vi "prima_apl_v0.vi"() -> ()   [LabVIEW 2009]
panel:
  out "Array":bool[](array[boolean])
  out "Numeric 8":dbl
  out "Numeric 7":dbl
  out "Numeric 6":dbl
  out "Numeric 5":dbl
  out "Numeric 4":dbl
  out "Numeric 3":dbl
  out "Numeric 2":dbl
  out "Numeric1":dbl
  out "Boolean 8":bool
  out "Boolean 7":bool
  out "Boolean 6":bool
  out "Boolean 5":bool
  out "Boolean 4":bool
  out "Boolean 3":bool
  out "Boolean 2":bool
  out "Boolean1":bool
  in  "Numeric 9":u8
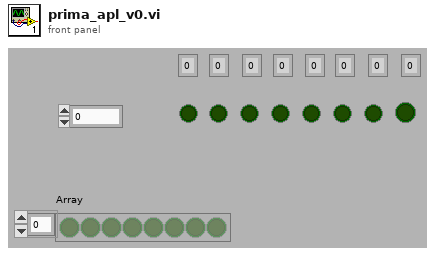
[diagram p1: front panel]
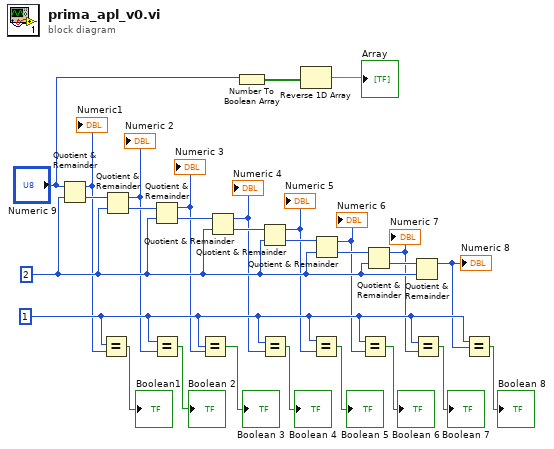
[diagram p0: block diagram]
diagram:
  w11 = 2
  w23 = 1
  n1 = Quotient & Remainder(x="Numeric 9", y=w11) -> (x-y*floor(x/y)=w4:i32, floor(x/y)=w14:i32)
  "Numeric1" <- w4
  n2 = Equal?(x=w23, y=w4) -> (x = y?=→"Boolean1":bool)
  n3 = Quotient & Remainder(x=w14, y=w11) -> (x-y*floor(x/y)=w5:i32, floor(x/y)=w13:i32)
  "Numeric 2" <- w5
  n4 = Quotient & Remainder(x=w13, y=w11) -> (x-y*floor(x/y)=w6:i32, floor(x/y)=w12:i32)
  "Numeric 3" <- w6
  n5 = Equal?(x=w23, y=w5) -> (x = y?=→"Boolean 2":bool)
  n6 = Equal?(x=w23, y=w6) -> (x = y?=→"Boolean 3":bool)
  n7 = Quotient & Remainder(x=w12, y=w11) -> (x-y*floor(x/y)=w7:i32, floor(x/y)=w15:i32)
  "Numeric 4" <- w7
  n8 = Number To Boolean Array(number="Numeric 9") -> (Boolean array=w2:bool[])
  n9 = Quotient & Remainder(x=w15, y=w11) -> (x-y*floor(x/y)=w8:i32, floor(x/y)=w16:i32)
  "Numeric 5" <- w8
  n10 = Equal?(x=w23, y=w7) -> (x = y?=→"Boolean 4":bool)
  n11 = Reverse 1D Array(array=w2) -> (reversed array=→"Array":bool[])
  n12 = Equal?(x=w23, y=w8) -> (x = y?=→"Boolean 5":bool)
  n13 = Quotient & Remainder(x=w16, y=w11) -> (x-y*floor(x/y)=w9:i32, floor(x/y)=w17:i32)
  "Numeric 6" <- w9
  n14 = Equal?(x=w23, y=w9) -> (x = y?=→"Boolean 6":bool)
  n15 = Quotient & Remainder(x=w17, y=w11) -> (x-y*floor(x/y)=w10:i32, floor(x/y)=w18:i32)
  "Numeric 7" <- w10
  n16 = Quotient & Remainder(x=w18, y=w11) -> (x-y*floor(x/y)=w22:i32)  [unwired: 1 out]
  "Numeric 8" <- w22
  n17 = Equal?(x=w23, y=w10) -> (x = y?=→"Boolean 7":bool)
  n18 = Equal?(x=w23, y=w22) -> (x = y?=→"Boolean 8":bool)
